vi "GetAttribute.vi"(8 "error in (no error)":errorcluster, 11 "Data_Pupil in":refnum<class "Data_Pupil.lvclass">) -> (0 "error out":errorcluster, 2 "Attribute":T1, 3 "Data_Pupil out":refnum<class "Data_Pupil.lvclass">)   [LabVIEW 2020, in "Data_Pupil.lvclass"]
uses:
  Data_Pupil.lvclass
  Attribute.vi
  Data_Pupil.lvclass/Data_Pupil.ctl
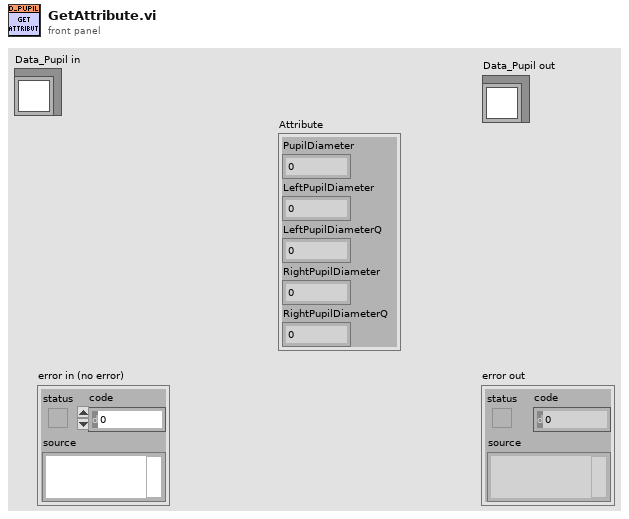
[diagram p1: front panel]
types:
  T1 = typedef "Data_Pupil.lvclass/Attribute.vi" = cluster{"PupilDiameter":dbl, "LeftPupilDiameter":dbl, "LeftPupilDiameterQ":dbl, "RightPupilDiameter":dbl, "RightPupilDiameterQ":dbl}
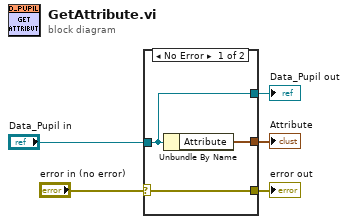
[diagram p0: block diagram]
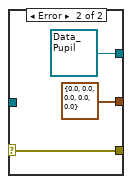
[diagram p2: hidden frame]
diagram:
  n1 = case shown="No Error" "error in (no error)" {
    selector: "error in (no error)" -> [w8 w11]
    tunnel: [w8 w11] -> w4
    tunnel: [w7 refnum<class "Data_Pupil.lvclass"> refnum ("Data_Pupil_Diameter in")] -> w3
    tunnel: "Data_Pupil in" -> [w7 _]
    tunnel: [w6 T1 {"PupilDiameter"=0.0, "LeftPupilDiameter"=0.0, "LeftPupilDiameterQ"=0.0, "RightPupilDiameter"=0.0, "RightPupilDiameterQ"=0.0} ("Attribute")] -> w1
    frame No Error {
      n2 = Unbundle By Name(w7) -> ("Attribute"=w6:T1)
    }
    frame Error {
    }
  }
  "error out" <- w4
  "Data_Pupil out" <- w3
  "Attribute" <- w1
